vi "MH_T2 Read Acq Queue.vi"() -> ()   [LabVIEW 2019]
uses:
  <userlib>/MultiHarp150/T2Lib/MH_T2QMessage.ctl
  <userlib>/MultiHarp150/T2Lib/MH_T2DeltaQMessage.ctl
  <userlib>/MultiHarp150/T2Lib/MH_ResizeBuffer.vi
panel:
  out "SpBufSze":i32=1000000
  in  "Dbuffsize":i32=10
  out "Done":bool
  out "TotalRec":i32
  out "TotalTime":u32
  in  "stop":bool
  out "sortie d'erreur":errorcluster caption="ErrorOut"
  out "RollOver":bool
  in  "StBufSze":i32=1000000
  in  "entrée d'erreur":errorcluster caption="ErrorIn"
  in  "WIndowW":i32
  in  "Save Data":bool
  in  "StopCh":u32=2
  in  "StartCh":u32=1
  in  "refnum":refnum<file>
  out "DeltaT":u32[](array[numeric])
  out "nActual":i32[](array[numeric])
  out "En Attente":i32[](array[numeric])
  out "Tableau":u64[][](array[numeric])
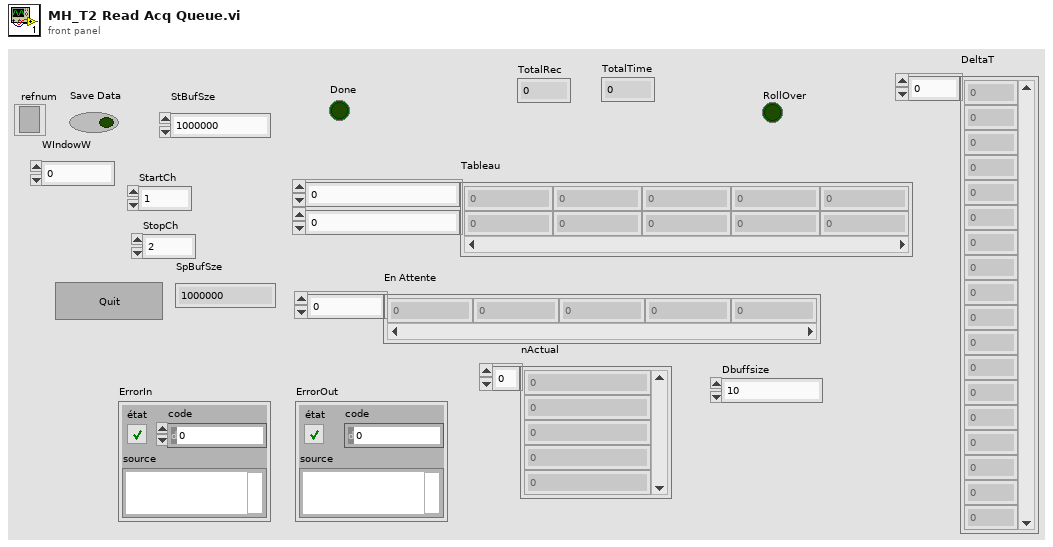
[diagram p1: front panel]
types:
  T1 = typedef "MH_T2DeltaQMessage.ctl" = cluster{"Message":string, "buffer":i32[], "Code":i32, "nactual":i32}
  T2 = typedef "MH_T2QMessage.ctl" = cluster{"Message":string, "buffer":u32[], "Code":i32, "nactual":i32}
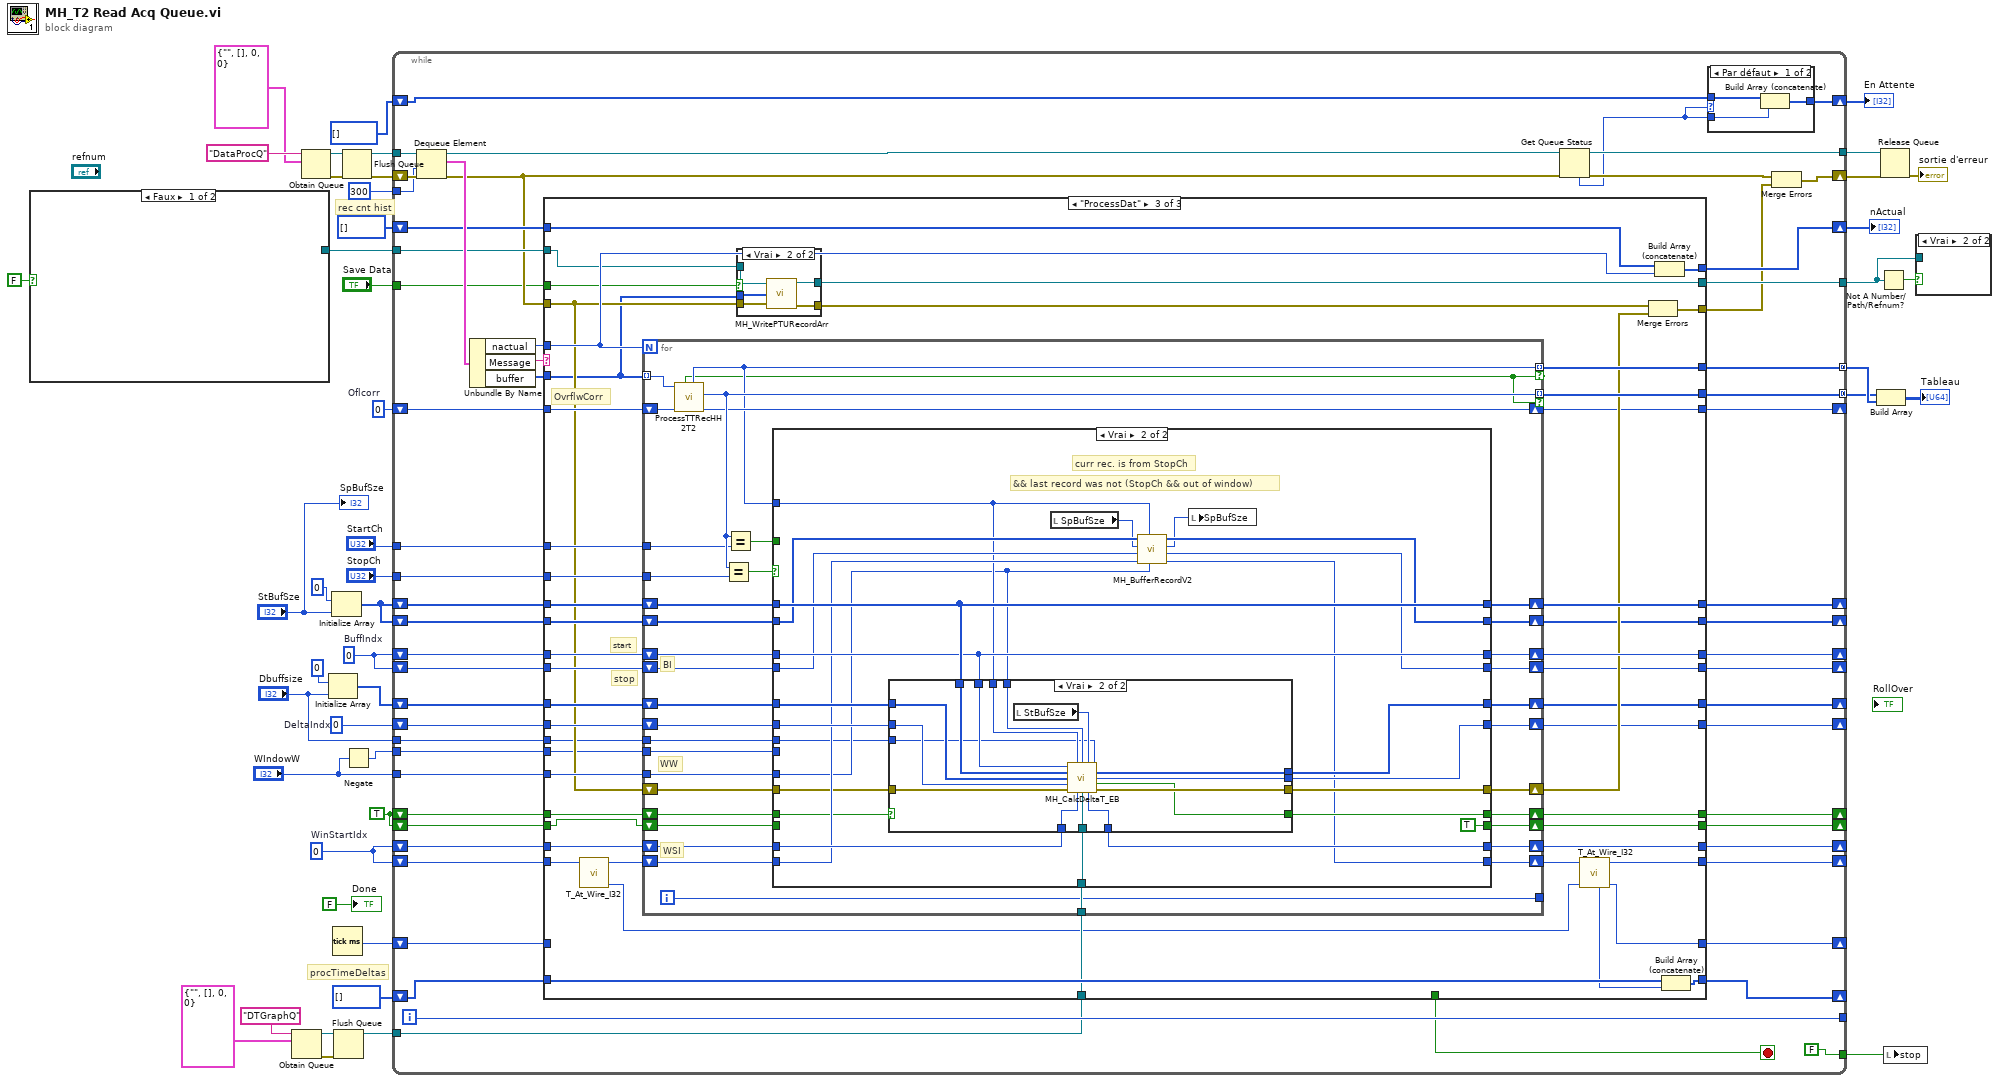
[diagram p0: block diagram]
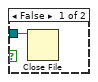
[diagram p2: hidden frame]
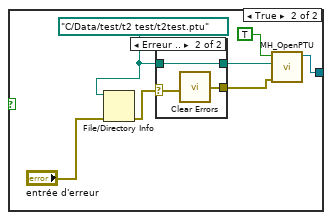
[diagram p3: hidden frame]
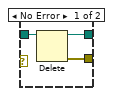
[diagram p4: hidden frame]
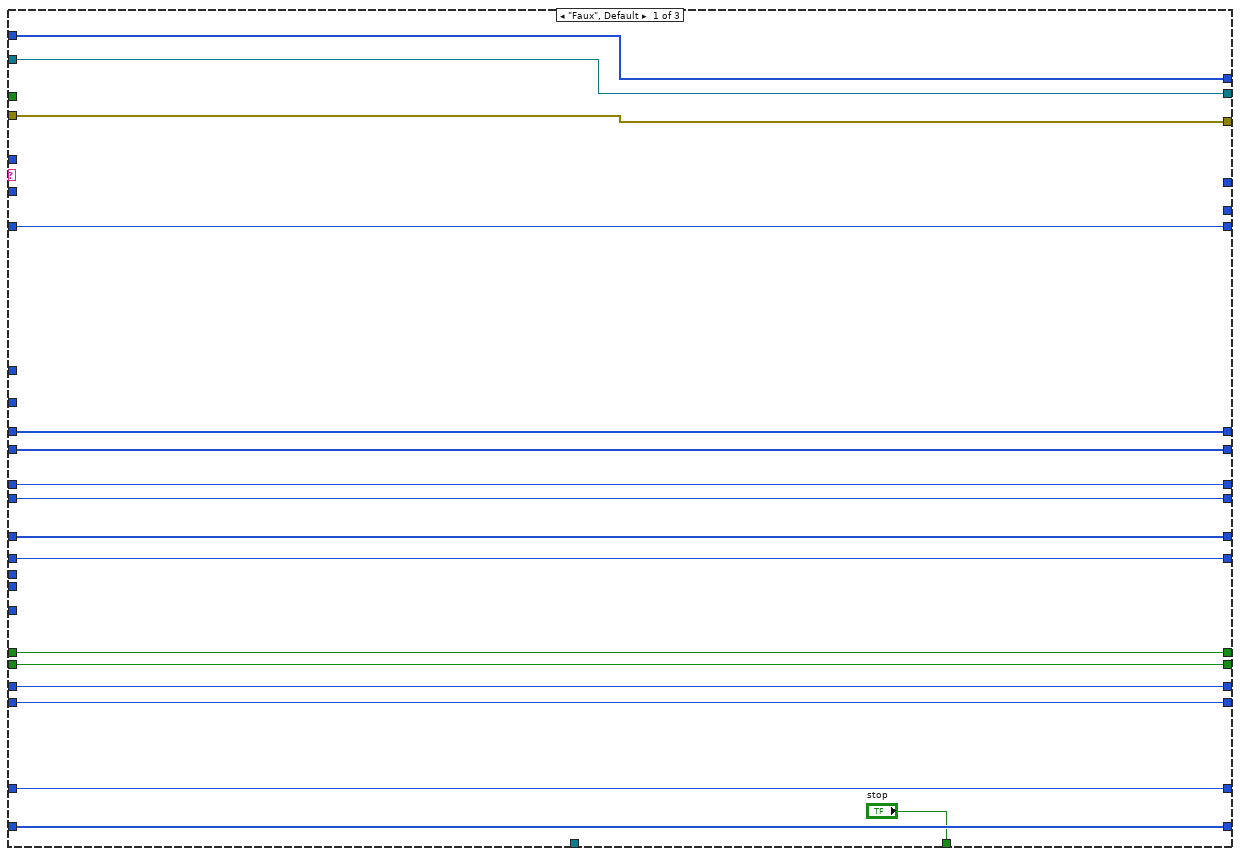
[diagram p6: hidden frame]
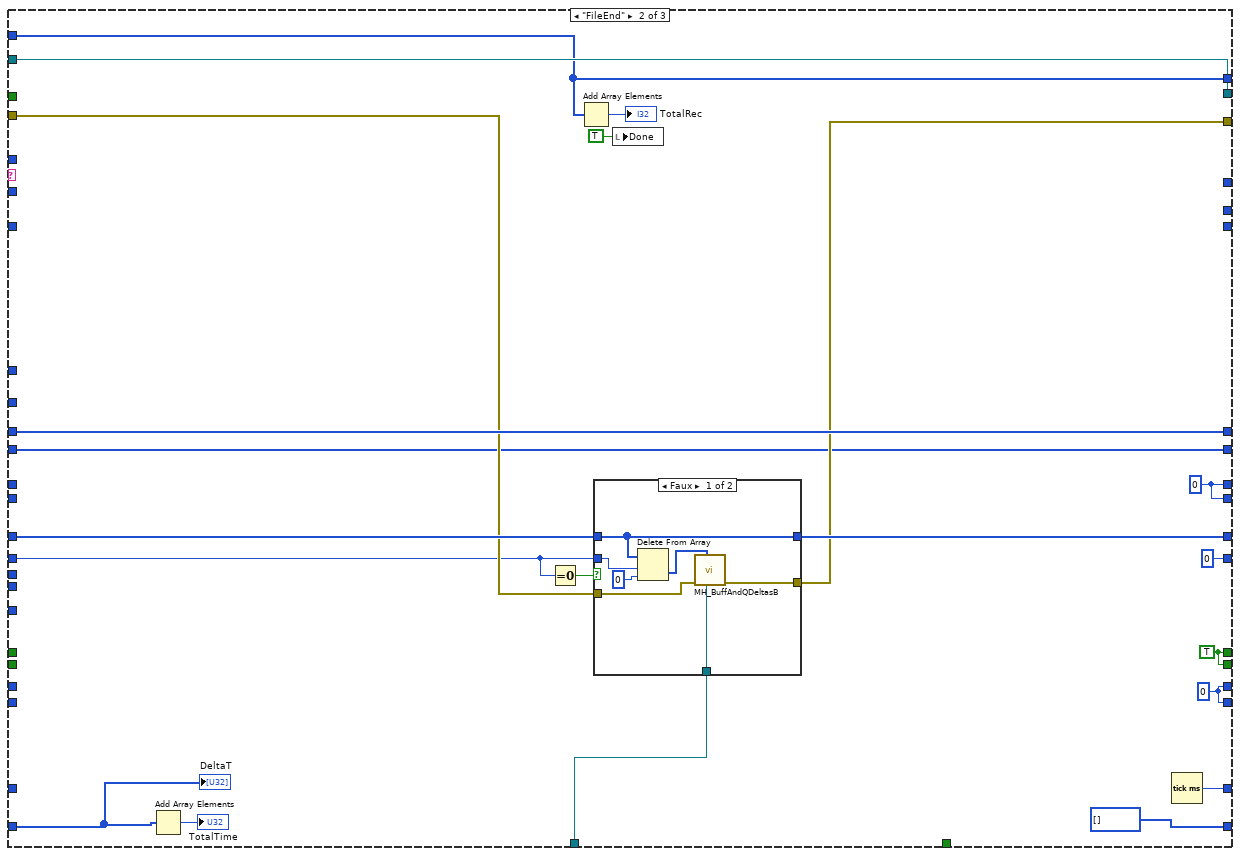
[diagram p7: hidden frame]
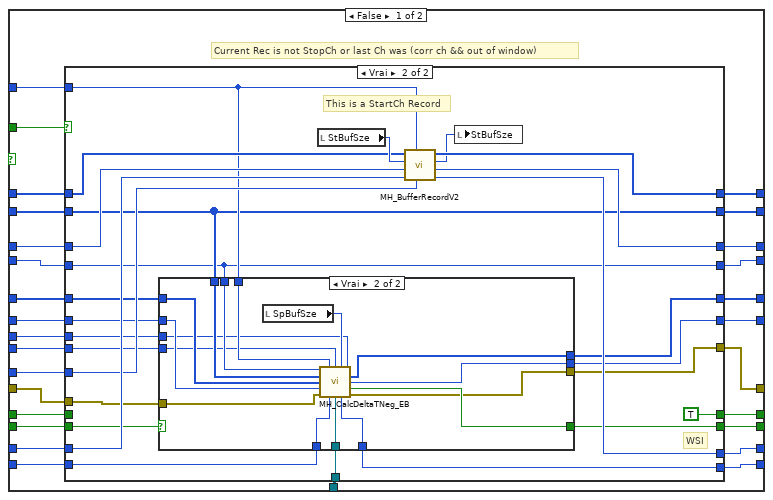
[diagram p10: hidden frame]
diagram:
  w11 = 0  # DeltaIndx
  w6 = TRUE
  w7 = 0  # WinStartIdx
  w8 = 0  # BuffIndx
  w44 = u64 0  # Oflcorr
  # "procTimeDeltas"
  # "rec cnt hist"
  n1 = case shown="Faux" FALSE {
    tunnel: [_ w52] -> w32
    frame False {
    }
    frame True {
      w49 = path "C:/Data/test/t2 test/t2test.ptu" ("chemin sélectionné")
      n2 = File/Directory Info(path=w49, error in="entrée d'erreur") -> (error out=w48:errorcluster)  [unwired: 6 out]
      n3 = case shown="Erreur .." w48 {
        selector: w48 -> [_ w58]
        tunnel: w49 -> [w56 w59]
        tunnel: [w55 w59] -> w51
        tunnel: [w54 w57] -> w50
        frame No Error {
          n4 = Delete(path (use dialog)=w56) -> (deleted path=w55:path, error out=w54:errorcluster)  [unwired: 4 in, 1 out]
        }
        frame Error {
          n5 = call <vilib>:"Clear Errors.vi"("error in (no error)"=w58) -> ("error out"=w57:errorcluster)  [unwired: 5 in, 1 out]
        }
      }
      n6 = call <userlib>:"MH_OpenPTU.vi"("ErrorIn"=w50, "chemin sélectionné"=w51, "WriteMode"=TRUE) -> ("refnum en sortie"=w52:refnum<file>)  [unwired: 6 in, 2 out]
    }
  }
  n7 = Obtain Queue(name (unnamed)="DTGraphQ" ("nom (aucun)"), element data type=T1 {"Message"="", "buffer"=[], "Code"=0, "nactual"=0} ("ClassQueue")) -> (queue out=w13:refnum<queue>, error out=w14:errorcluster)  [unwired: 3 in, 1 out]
  n8 = Obtain Queue(name (unnamed)="DataProcQ" ("nom (aucun)"), element data type=T2 {"Message"="", "buffer"=[], "Code"=0, "nactual"=0} ("ClassQueue")) -> (queue out=w18:refnum<queue>, error out=w15:errorcluster)  [unwired: 3 in, 1 out]
  n9 = Initialize Array(0 ("truetime"), "Dbuffsize") -> (w19:i32[])
  n10 = Initialize Array(u64 0 ("truetime"), "StBufSze") -> (w9:u64[])
  n11 = Tick Count (ms)() -> (millisecond timer value=w37:u32)
  n12 = Flush Queue(queue=w13, error in (no error)=w14) -> (queue out=w22:refnum<queue>)  [unwired: 2 out]
  n13 = Flush Queue(queue=w18, error in (no error)=w15) -> (queue out=w17:refnum<queue>, error out=w16:errorcluster)  [unwired: 1 out]
  n14 = Negate(x="WIndowW") -> (-x=w1:i32)
  n15 = while {
    tunnel: w17 -> [w116]
    shift-right: [w94] -> w43
    shift-left: w16 -> [w117]
    shift-right: [w114] -> _
    shift-left: w44 -> [w115]
    tunnel: [w113] -> w40 mode=concatenating
    tunnel: [w110] -> _
    tunnel: [w106] -> w42
    tunnel: [w105] -> w39 mode=concatenating
    shift-right: [w103] -> _
    shift-left: w37 -> [w104]
    shift-right: [w101] -> _
    shift-left: u32[] [] ("DeltaT") -> [w102]
    shift-right: [w99] -> w34
    shift-left: i32[] [] ("DeltaT") -> [w100]
    shift-right: [w98] -> w41
    shift-left: i32[] [] ("DeltaT") -> [w97]
    tunnel: w32 -> [w96]
    tunnel: [w93] -> w24
    tunnel: "Save Data" -> [w92]
    shift-right: [w87] -> _
    shift-left: w9 -> [w91]
    shift-right: [w89] -> _
    shift-left: w8 -> [w90]
    tunnel: "StopCh" -> [w88]
    shift-right: [w83] -> _
    shift-left: w7 -> [w86]
    tunnel: "WIndowW" -> [w85]
    tunnel: 300 ("timeout en ms (-1)") -> [w84]
    tunnel: w22 -> [w81]
    shift-right: [w79] -> _
    shift-left: w6 -> [w78]
    shift-right: [w63] -> _
    shift-left: w19 -> [w77]
    tunnel: [FALSE] -> w12
    shift-right: [w72] -> _
    shift-left: w11 -> [w73]
    shift-right: [w66] -> _
    shift-left: w9 -> [w71]
    shift-right: [w67] -> _
    shift-left: w8 -> [w70]
    shift-right: [w68] -> _
    shift-left: w7 -> [w69]
    shift-right: [w64] -> _
    shift-left: w6 -> [w65]
    tunnel: "StartCh" -> [w62]
    tunnel: "Dbuffsize" -> [w61]
    tunnel: w1 -> [w60]
    i -> [w110]
    stop <- w76 stop-if-true
    n16 = Dequeue Element(queue=w116, timeout in ms (-1)=w84, error in (no error)=w117) -> (queue out=w108:refnum<queue>, element=w112:T2, error out=w95:errorcluster)  [unwired: 1 out]
    n17 = Unbundle By Name(w112) -> ("nactual"=w82:i32, "Message"=w109:string, "buffer"=w111:u32[])
    n18 = case shown="\"ProcessDat\"" w109 {
      tunnel: w115 -> [w138 _ w216]
      tunnel: [w138 _ w169] -> w114
      tunnel: [_ _ w215] -> w113
      tunnel: w111 -> [_ _ w182]
      tunnel: [_ _ w214] -> w105
      tunnel: w104 -> [w137 _ _]
      tunnel: [w136 u32[] [] ("DeltaT") w212] -> w101
      tunnel: [w137 w157 w172] -> w103
      tunnel: w102 -> [w136 w155 w213]
      tunnel: w100 -> [w135 w152 w211]
      tunnel: [w135 w152 w210] -> w99
      tunnel: w96 -> [w122 w159 w185]
      tunnel: w95 -> [w131 w146 w183]
      tunnel: [w122 w159 w179] -> w93
      tunnel: w92 -> [_ _ w184]
      tunnel: w91 -> [w133 w158 w200]
      tunnel: w90 -> [w134 _ w201]
      tunnel: [w134 w141 w208] -> w89
      tunnel: w88 -> [_ _ w209]
      tunnel: [w133 w158 w207] -> w87
      tunnel: w86 -> [w132 _ w195]
      tunnel: w85 -> [_ _ w206]
      tunnel: [w132 w142 w205] -> w83
      tunnel: w82 -> [_ _ w204]
      tunnel: w81 -> [_ w143 w203]
      tunnel: [w131 w147 w181] -> w80
      tunnel: [w130 w139 w199] -> w79
      tunnel: w78 -> [w130 _ w198]
      tunnel: w77 -> [w129 w149 w197]
      tunnel: [w129 w148 w196] -> w63
      tunnel: ["stop" _ _] -> w76
      tunnel: w73 -> [w127 w145 w194]
      tunnel: [w127 0 w193] -> w72
      tunnel: w71 -> [w124 w140 w192]
      tunnel: w70 -> [w125 _ w191]
      tunnel: w69 -> [w126 _ w176]
      tunnel: [w126 w142 w173] -> w68
      tunnel: [w125 w141 w190] -> w67
      tunnel: [w124 w140 w189] -> w66
      tunnel: w65 -> [w123 _ w188]
      tunnel: [w123 w139 w187] -> w64
      tunnel: w62 -> [_ _ w186]
      tunnel: w61 -> [_ _ w178]
      tunnel: w60 -> [_ _ w177]
      frame "Faux", Default {
      }
      frame "FileEnd" {
        w139 = TRUE
        w142 = 0 ("WinStartIdx")
        w141 = 0 ("BuffIndx")
        n19 = Add Array Elements(numeric array=w155) -> (sum=→"TotalTime":u32)
        n20 = Equal To 0?(x=w145) -> (x = 0?=w144:bool)
        n21 = Add Array Elements(numeric array=w152) -> (sum=→"TotalRec":i32)
        n22 = case shown="Faux" w144 {
          tunnel: w149 -> [w163 w168]
          tunnel: [w163 w168] -> w148
          tunnel: [w166 w167] -> w147
          tunnel: w146 -> [w165 w167]
          tunnel: w145 -> [w162 _]
          tunnel: w143 -> [w164 _]
          frame False {
            n23 = Delete From Array(array=w163, length=w162, index=0 ("indice")) -> (deleted portion=w160:i32[])  [unwired: 1 out]
            n24 = call <userlib>:"MH_BuffAndQDeltasB.vi"("queue out"=w164, "DeltasBuffer"=w160, "erroIn"=w165) -> ("error out"=w166:errorcluster)  [unwired: 8 in]
          }
          frame True {
          }
        }
        n25 = local write "Done"(TRUE ("Done")) -> ()
        n26 = Tick Count (ms)() -> (millisecond timer value=w157:u32)
        "DeltaT" <- w155
      }
      frame "ProcessDat" {
        # "stop"
        # "start"
        # "OvrflwCorr"
        n27 = call <userlib>:"T_At_Wire_I32.vi"("I32"=w176) -> ("Clock(ms)"=w170:u32, "I32 Out"=w175:i32)  [unwired: 8 in, 1 out]
        n28 = for {
          N: w204 -> [_]
          tunnel: [w248] -> w215 mode=indexing if=w240
          tunnel: w182 -> [w259] mode=indexing
          tunnel: [w258] -> w214 mode=indexing if=w240
          shift-right: [w245] -> w207
          shift-left: w200 -> [w249]
          shift-right: [w246] -> w208
          shift-left: w201 -> [w247]
          tunnel: w209 -> [w257]
          tunnel: w206 -> [w256]
          shift-right: [w255] -> w169
          shift-left: w216 -> [w260]
          shift-right: [w254] -> w205
          shift-left: w195 -> [w251]
          shift-right: [w252] -> w202
          shift-left: w183 -> [w226]
          tunnel: w203 -> [w253]
          shift-right: [w244] -> w199
          shift-left: w198 -> [w243]
          shift-right: [w241] -> w196
          shift-left: w197 -> [w242]
          shift-right: [w238] -> w193
          shift-left: w194 -> [w239]
          tunnel: w186 -> [w237]
          shift-right: [w234] -> w189
          shift-left: w192 -> [w235]
          tunnel: [w236] -> _
          shift-right: [w230] -> w190
          shift-left: w191 -> [w233]
          shift-right: [w231] -> w174
          shift-left: w175 -> [w232]
          shift-right: [w227] -> w187
          shift-left: w188 -> [w228]
          tunnel: w178 -> [w225]
          tunnel: w177 -> [w224]
          i -> [w236]
          # "WW"
          # "BI"
          # "WSI"
          n29 = call <userlib>:"ProcessTTRecHH2T2.vi"("oflcorr_in"=w260, "rawbits"=w259) -> ("oflcorr_out"=w255:u64, "channel"=w258:u32, "truetime"=w248:u64, "is_photon"=w240:bool)  [unwired: 4 in, 2 out]
          n30 = Equal?(x=w258, y=w257) -> (x = y?=w229:bool)
          n31 = Equal?(x=w258, y=w237) -> (x = y?=w250:bool)
          n32 = case shown="Vrai" w229 {
            tunnel: w249 -> [w287 w371]
            tunnel: w251 -> [w283 w369]
            tunnel: w247 -> [w285 w370]
            tunnel: w256 -> [w281 w354]
            tunnel: [w280 w368] -> w254
            tunnel: w253 -> [w267 w347]
            tunnel: [w273 w362] -> w252
            tunnel: w250 -> [w286 _]
            tunnel: w248 -> [w282 w355]
            tunnel: [w284 w370] -> w246
            tunnel: [w288 w371] -> w245
            tunnel: [w279 w365] -> w244
            tunnel: w243 -> [w278 w351]
            tunnel: w242 -> [w263 w367]
            tunnel: [w270 w364] -> w241
            tunnel: w239 -> [w272 w366]
            tunnel: [w271 w363] -> w238
            tunnel: w235 -> [w277 w361]
            tunnel: [w268 w360] -> w234
            tunnel: w233 -> [w276 w359]
            tunnel: w232 -> [w275 w358]
            tunnel: [w274 w353] -> w231
            tunnel: [w269 w352] -> w230
            tunnel: w228 -> [w266 _]
            tunnel: [w265 TRUE ("NewDelta")] -> w227
            tunnel: w226 -> [w264 w349]
            tunnel: w225 -> [w262 w348]
            tunnel: w224 -> [w261 _]
            frame False {
              # "Current Rec is not StopCh or last Ch was (corr ch && out of window)"
              n33 = case shown="Vrai" w286 {
                tunnel: w287 -> [w298 w317]
                tunnel: w282 -> [_ w312]
                tunnel: w285 -> [w299 w320]
                tunnel: [w299 w324] -> w284
                tunnel: [w298 w323] -> w288
                tunnel: w283 -> [w297 w321]
                tunnel: w281 -> [_ w314]
                tunnel: [w297 w322] -> w280
                tunnel: [w296 TRUE] -> w279
                tunnel: w278 -> [w296 _]
                tunnel: w277 -> [w291 w309]
                tunnel: w276 -> [w292 w308]
                tunnel: w275 -> [w293 w316]
                tunnel: [w293 w315] -> w274
                tunnel: [w289 w313] -> w273
                tunnel: w272 -> [w294 w304]
                tunnel: [w294 w303] -> w271
                tunnel: [w295 w302] -> w270
                tunnel: w263 -> [w295 w311]
                tunnel: [w292 w308] -> w269
                tunnel: [w291 w309] -> w268
                tunnel: w267 -> [_ w310]
                tunnel: w266 -> [w290 w307]
                tunnel: [w290 w306] -> w265
                tunnel: w264 -> [w289 w305]
                tunnel: w262 -> [_ w301]
                tunnel: w261 -> [_ w300]
                frame False {
                  # "could be sync or non-relevant channel"
                }
                frame True {
                  # "This is a StartCh Record"
                  # "WSI"
                  n34 = case shown="Vrai" w307 {
                    selector: w307 -> [w330 _]
                    tunnel: w309 -> [_ w346]
                    tunnel: w308 -> [_ w345]
                    tunnel: w316 -> [w329 w344]
                    tunnel: [w329 w340] -> w315
                    tunnel: w311 -> [w327 w339]
                    tunnel: w304 -> [w326 w338]
                    tunnel: w305 -> [w328 w337]
                    tunnel: [w330 w341] -> w306
                    tunnel: [w327 w335] -> w302
                    tunnel: [w326 w334] -> w303
                    tunnel: w310 -> [_ w336]
                    tunnel: [w328 w333] -> w313
                    tunnel: w312 -> [_ w342]
                    tunnel: w301 -> [_ w332]
                    tunnel: w300 -> [_ w331]
                    frame False {
                    }
                    frame True {
                      n35 = local read "SpBufSze"() -> (w343:i32)
                      n36 = call <userlib>:"MH_CalcDeltaTNeg_EB.vi"("Buffindex"=w345, "TrueTime"=w342, "WIndowW"=w331, "Buffsize"=w343, "DBuffSize"=w332, "Data In"=w346, "DeltasBuffer"=w339, "Deltaindex"=w338, "error In"=w337, "WinIndex"=w344, "queue out"=w336) -> ("DeltasBufferOut"=w335:i32[], "DeltaIndexOut"=w334:i32, "NewDelta"=w341:bool, "WinIndexOut"=w340:i32, "Error Out"=w333:errorcluster)
                    }
                  }
                  n37 = local read "StBufSze"() -> (w319:i32)
                  n38 = call <userlib>:"MH_BufferRecordV2.vi"("WindowWidth"=w314, "truetime"=w312, "WinIndex"=w321, "Buffindex"=w320, "Buffsize"=w319, "Buffer"=w317) -> ("WinIndexOut"=w322:i32, "BuffIndexOut"=w324:i32, "NewBuffsize"=w318:i32, "tableau (n rotations)"=w323:u64[])  [unwired: 2 in]
                  n39 = local write "StBufSze"(w318) -> ()
                }
              }
            }
            frame True {
              # "&& last record was not (StopCh && out of window)"
              # "curr rec. is from StopCh"
              n40 = case shown="Vrai" w351 {
                selector: w351 -> [w376 _]
                tunnel: w371 -> [_ w392]
                tunnel: w370 -> [_ w391]
                tunnel: w369 -> [w372 w387]
                tunnel: [w372 w388] -> w368
                tunnel: w367 -> [w374 w386]
                tunnel: w366 -> [w373 w385]
                tunnel: w349 -> [w375 w380]
                tunnel: [w376 w377] -> w365
                tunnel: [w374 w379] -> w364
                tunnel: [w373 w378] -> w363
                tunnel: w347 -> [_ w383]
                tunnel: [w375 w382] -> w362
                tunnel: w355 -> [_ w389]
                tunnel: w354 -> [_ w384]
                tunnel: w348 -> [_ w381]
                frame False {
                }
                frame True {
                  n41 = local read "StBufSze"() -> (w390:i32)
                  n42 = call <userlib>:"MH_CalcDeltaT_EB.vi"("Buffindex"=w391, "TrueTime"=w389, "WIndowW"=w384, "Buffsize"=w390, "DBuffSize"=w381, "Data In"=w392, "DeltasBuffer"=w386, "Deltaindex"=w385, "error In"=w380, "WinIndex"=w387, "queue out"=w383) -> ("DeltasBufferOut"=w379:i32[], "DeltaIndexOut"=w378:i32, "NewDelta"=w377:bool, "WinIndexOut"=w388:i32, "Error Out"=w382:errorcluster)
                }
              }
              n43 = local read "SpBufSze"() -> (w357:i32)
              n44 = call <userlib>:"MH_BufferRecordV2.vi"("WindowWidth"=w354, "truetime"=w355, "WinIndex"=w358, "Buffindex"=w359, "Buffsize"=w357, "Buffer"=w361) -> ("WinIndexOut"=w353:i32, "BuffIndexOut"=w352:i32, "NewBuffsize"=w356:i32, "tableau (n rotations)"=w360:u64[])  [unwired: 2 in]
              n45 = local write "SpBufSze"(w356) -> ()
            }
          }
        }
        n46 = case shown="Vrai" w184 {
          tunnel: w185 -> [w217 w223]
          tunnel: w183 -> [w218 w222]
          tunnel: [w217 w221] -> w179
          tunnel: [w218 w220] -> w180
          tunnel: w182 -> [_ w219]
          frame False {
          }
          frame True {
            n47 = call <userlib>:"MH_WritePTURecordArr.vi"("refnum"=w223, "TTTR Records"=w219, "error in"=w222) -> ("refnum en sortie"=w221:refnum<file>, "error out"=w220:errorcluster)  [unwired: 6 in]
          }
        }
        n48 = call <userlib>:"T_At_Wire_I32.vi"("InitClock(ms)"=w170, "I32"=w174) -> ("Clock(ms)"=w172:u32, "I32 Out"=w173:i32, "Delta(ms)"=w171:u32)  [unwired: 7 in]
        n49 = Merge Errors(w180, w202) -> (w181:errorcluster)
        n50 = Build Array (concatenate)(w211, w204) -> (w210:i32[])
        n51 = Build Array (concatenate)(w213, w171) -> (w212:u32[])
      }
    }
    n52 = Get Queue Status(queue=w108, error in (no error)=w95) -> (queue out=w106:refnum<queue>, error out=w107:errorcluster, # elements in queue=w74:i32)  [unwired: 1 in, 5 out]
    n53 = case shown="Par défaut" w74 {
      tunnel: w74 -> [w120 _]
      tunnel: [w119 w121] -> w98
      tunnel: w97 -> [w118 w121]
      frame Default {
        n54 = Build Array (concatenate)(w118, w120) -> (w119:i32[])
      }
      frame 0 {
      }
    }
    n55 = Merge Errors(w107, w80) -> (w94:errorcluster)
  }
  "En Attente" <- w41
  "nActual" <- w34
  n56 = Build Array(w39, w40) -> (→"Tableau":u64[][])
  n57 = Not A Number/Path/Refnum?(number/path/refnum=w24) -> (NaN/Path/Refnum?=w23:bool)
  n58 = Release Queue(queue=w42, error in (no error)=w43) -> (error out=→"sortie d'erreur":errorcluster)  [unwired: 1 in, 2 out]
  n59 = local write "stop"(w12) -> ()
  n60 = case shown="Vrai" w23 {
    tunnel: w24 -> [w393 _]
    frame False {
      n61 = Close File(refnum=w393) -> ()  [unwired: 1 in, 2 out]
    }
    frame True {
    }
  }
  "Done" <- FALSE
  "SpBufSze" <- "StBufSze"
